vi "PXI Stop AI.vi"(8 "error in":errorcluster) -> (0 "error out":errorcluster)   [LabVIEW 2015]
uses:
  PXI Globals.vi
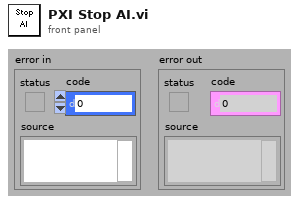
[diagram p1: front panel]
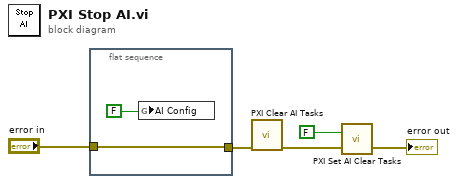
[diagram p0: block diagram]
diagram:
  n1 = flat-sequence {
    tunnel: "error in" -> [w6]
    tunnel: [w6] -> w1
    frame #0 {
      n2 = global write "PXI Globals.vi" "AI Config"(FALSE) -> ()
    }
  }
  n3 = call "PXI Clear AI Tasks.vi"("error in"=w1) -> ("error out"=w4:errorcluster)  [unwired: 10 in]
  n4 = call "PXI Set AI Clear Tasks.vi"("error in (no error)"=w4, "AI ClearTasks"=FALSE) -> ("error out"=→"error out":errorcluster)  [unwired: 1 in]
